vi "ReadDMM_FGV.vi"(6 "Priority":bool, 8 "error in (no error)":errorcluster, 9 "Message Data":variant, 10 "Message":string) -> (0 "error out":errorcluster)   [LabVIEW 2024, in "DMM6500.lvlib"]
doc: "ThisVI\n------------------------------\nEnqueue Message\n------------------------------\n-Enqueue the message in message queue.\n-set Priority to true to enqueue at oposite end"
uses:
  DMM6500.lvlib
  PrivateControls/DMM6500_FGV_Queue_Control.ctl
  support/Message Queue/DMM6500_Message Cluster.ctl
  support/Message Queue/DMM6500 Message Queue.lvlib
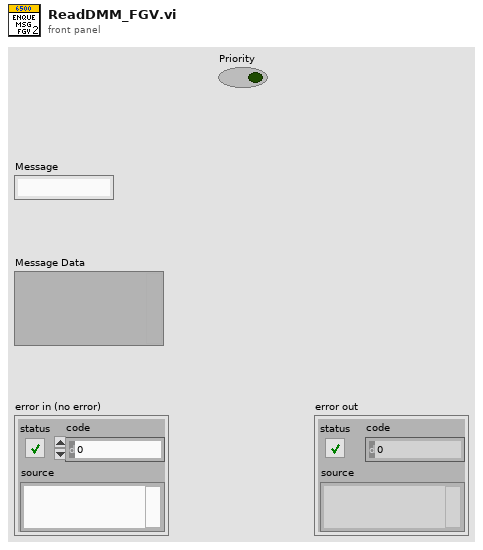
[diagram p1: front panel]
types:
  T1 = typedef "DMM6500.lvlib/DMM6500 Message Queue.lvlib/DMM6500_Message Cluster.ctl" = cluster{"Message":string, "Message Data":variant}
  T2 = typedef "DMM6500.lvlib/DMM6500_FGV_Queue_Control.ctl" = enum16{"Release", "Get", "Set"}
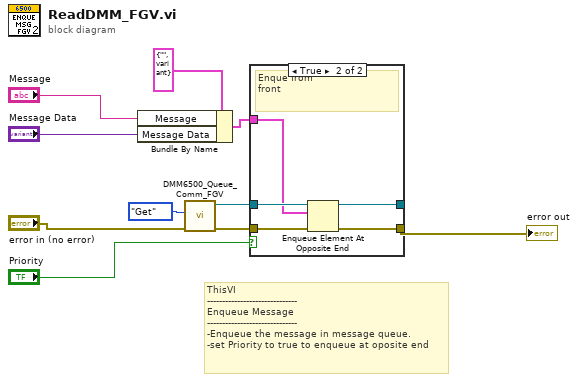
[diagram p0: block diagram]
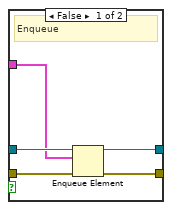
[diagram p2: hidden frame]
diagram:
  # "ThisVI\n------------------------------\nEnqueue Message\n------------------------------\n-Enqueue the message in message queue.\n-set Priority to true to enqueue at oposite end"
  n1 = Bundle By Name(cluster=T1 {"Message"="", "Message Data"=variant} ("element"), "Message"="Message", "Message Data"="Message Data") -> (w8:T1)
  n2 = call "DMM6500_Queue_Comm_FGV.vi"("error in (no error)"="error in (no error)", "Enum"=DMM6500_FGV_Queue_Control."Get") -> ("error Out"=w4:errorcluster, "queue Out"=w6:refnum<queue>)  [unwired: 8 in]
  n3 = case shown="True" "Priority" {
    tunnel: w4 -> [w15 w20]
    tunnel: [w14 w19] -> w5
    tunnel: w6 -> [w12 w18]
    tunnel: [w13 w17] -> _
    tunnel: w8 -> [w11 w16]
    frame False {
      # "Enqueue"
      n4 = Enqueue Element(queue=w12, element=w11, error in (no error)=w15) -> (queue out=w13:refnum<queue>, error out=w14:errorcluster)  [unwired: 1 in, 1 out]
    }
    frame True {
      # "Enque from\nfront"
      n5 = Enqueue Element At Opposite End(queue=w18, element=w16, error in (no error)=w20) -> (queue out=w17:refnum<queue>, error out=w19:errorcluster)  [unwired: 1 in, 1 out]
    }
  }
  "error out" <- w5
